vi "23384_Davis_Poku_Amankwa_Amankwa.DavisPoku.MNE1201.61_348261_1575301089.vi"() -> ()   [LabVIEW 2018]
panel:
  out "Total pay after 30 days in dollars":ext format="%#_13g"
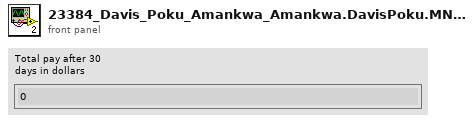
[diagram p1: front panel]
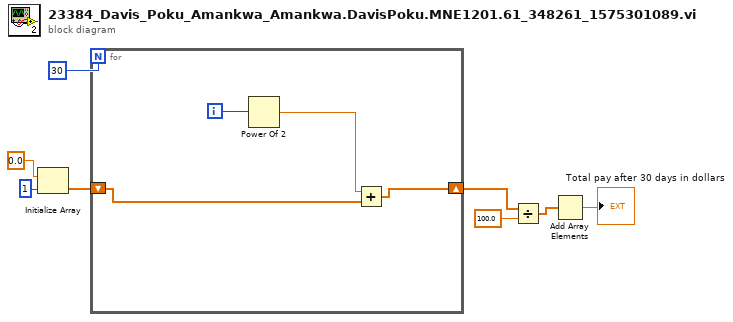
[diagram p0: block diagram]
diagram:
  n1 = Initialize Array(0.0 ("element"), 1) -> (w5:dbl[])
  n2 = for {
    N: 30 -> [_]
    shift-right: [w9] -> w6
    shift-left: w5 -> [w11]
    i -> [w12]
    n3 = Power Of 2(x=w12) -> (2^x=w10:dbl)
    n4 = Add(x=w10, y=w11) -> (x+y=w9:dbl[])
  }
  n5 = Divide(x=w6, y=100.0) -> (x/y=w3:dbl[])
  n6 = Add Array Elements(numeric array=w3) -> (sum=→"Total pay after 30 days in dollars":dbl)
